vi "Data-log-init.vi"() -> (2 "Data cluster":cluster{"Plant 1":T1, "Plant 2":T1}, 3 "Data array":dbl[][](array[numeric]))   [LabVIEW 2016]
uses:
  Plant-data.ctl
panel:
  in  "Data cluster":cluster{"Plant 2":T1, "Plant 1":T1}
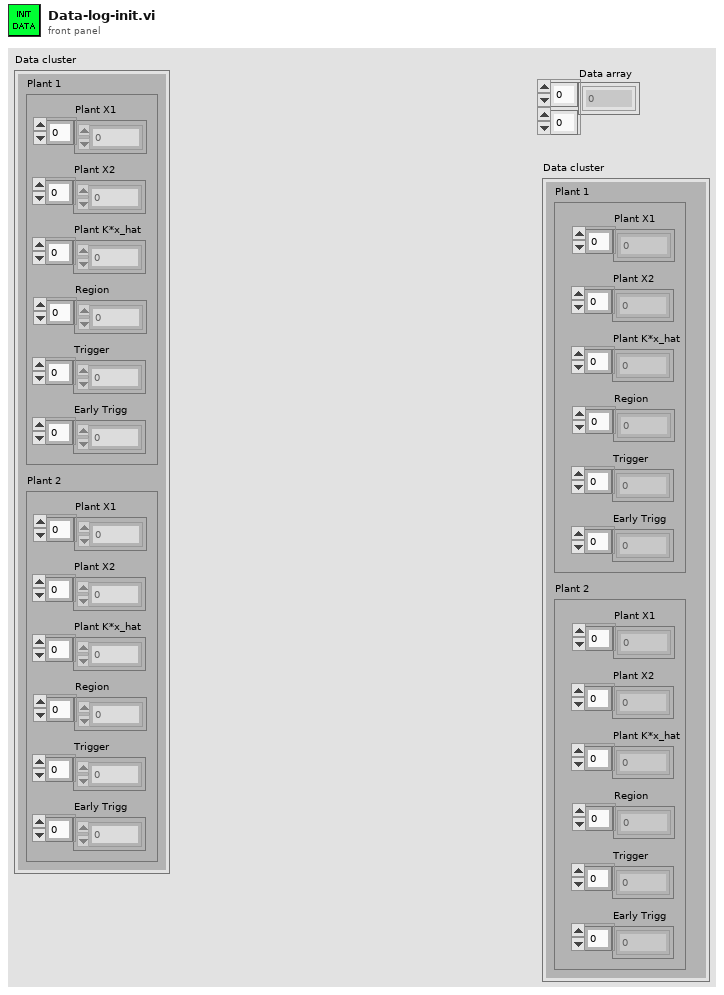
[diagram p1: front panel]
types:
  T1 = typedef "Plant-data.ctl" = cluster{"Plant X1 ":dbl[], "Plant X2":dbl[], "Plant K*x_hat":dbl[], "Region":i32[], "Trigger":i32[], "Early Trigg":i32[]}
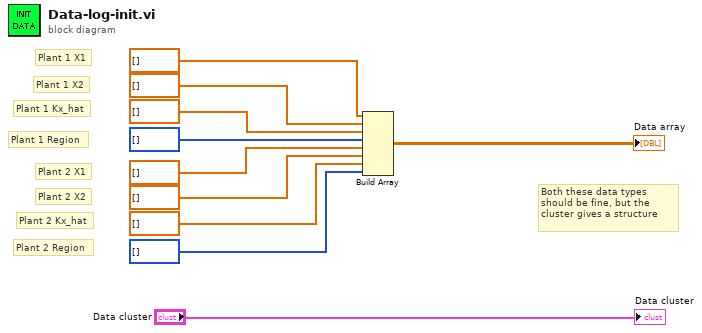
[diagram p0: block diagram]
diagram:
  # "Both these data types should be fine, but the cluster gives a structure"
  # "Plant 2 Region"
  # "Plant 1 Region"
  # "Plant 2 Kx_hat"
  # "Plant 2 X2"
  # "Plant 2 X1"
  # "Plant 1 Kx_hat"
  # "Plant 1 X2"
  # "Plant 1 X1"
  n1 = Build Array(dbl[] [], dbl[] [], dbl[] [], i32[] [], dbl[] [], dbl[] [], dbl[] [], i32[] []) -> (→"Data array":dbl[][])
  "Data cluster" <- "Data cluster"
